vi "4Pi Focus Lock_v1.vi"() -> ()   [LabVIEW 2016]
uses:
  4Pi Focus Lock Controls/4Pi Focus Lock - Notifier Type.ctl
  4Pi Focus Lock Controls/4Pi Focus Lock - Actions.ctl
  <vilib>/vision/Image Controls.llb/IMAQ Image.ctl
  Hardware Configuration/Hardware Configuration Controls/Device Type.ctl
  Hardware Configuration/Hardware Configuration Controls/Device Function.ctl
  Device Library/Cameras/Camera Controls/Generic Camera ROI.ctl
  Device Library/Cameras/Camera Controls/Generic Camera Actions.ctl
  Device Library/Stages/Stages Controls/Stage Actions.ctl
  <vilib>/addons/control/pid/pid.llb/PID (DBL).vi
  <vilib>/vision/NI_Vision_Development_Module.lvlib
  <vilib>/addons/control/pid/NI_PID_pid.lvlib
panel:
  in  "Z Drift Threshold (µm)":dbl=2.0
  in  "Z Move Limit (µm)":dbl=2.0
  out "Z Move":bool
  in  "Update Scale Factor":dbl=2.0
  out "dz (µm)":dbl format="%.2f"
  out "dt (s)":dbl format="%.3f"
  out "Measured Z (µm)":dbl=1.0 format="%.3g"
  out "Target Z (µm)":dbl=1.0 format="%.3g"
  out "Stage Position (µm)":dbl=1.0 format="%.2g"
  in  "Quit":bool
  in  "Sample Z Step No.":u32=2
  in  "Sample Z Step Size (µm)":dbl=2.0
  in  "D (Derivative)":dbl
  in  "I (Integral)":dbl
  in  "P (Proportional)":dbl=2.0
  in  "Set Camera ROI":bool
  out "Z Target and Fit Value (µm)":T1(graph)
  in  "Start Lock":bool
  # "PID Control Values"
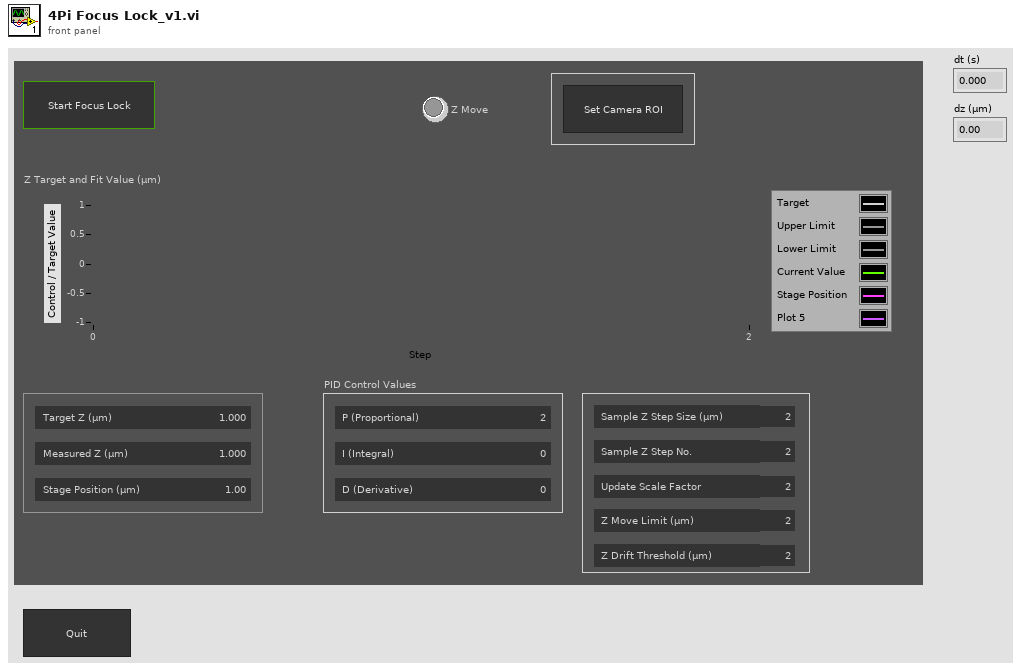
[diagram p1: front panel]
types:
  T1 = cluster{"Target 01":dbl, dbl, dbl, "Current 01":dbl, "Stage Position":dbl}
  T2 = typedef "4Pi Focus Lock - Actions.ctl" = enum16{"Idle", "Start Lock", "Restart Lock", "Get Target Position", "Get Ref Stack", "Cal Ref FFT", "Move To Init Z", "Start Primary Camera", "Get Current Position", "Get Current XY Position", "Get Current Position 1", "Get Actual Position", "Check Drift", "Move Z", "Update Plots", "Delay", "Abort", "Exit Loop", "Quit"}
  T3 = typedef "4Pi Focus Lock - Notifier Type.ctl" = cluster{"Actions":T2, "Z Drift Threshold":dbl, "Z Stage Move Limit (µm)":dbl, "Abort If Error":bool, "Z Correction Active":bool, "PID Values":dbl[], "Running?":bool, "Update Delay (ms)":i32, "Z Step Size (µm)":dbl, "Z Step No.":u32, "No. of Frames":u32, "Ref Stack (SGL)":T4[], "Cur Image (SGL)":T4, "CC Image (SGL) ":T4, "Sample Z (µm)":dbl[], "Initial Z Position (µm)":dbl, "Ref FFT Stack (CSG)":T4[], "Tmp Image FFT (CSG) ":T4[], "CC Image Max (SGL)":T4}
  T4 = typedef "IMAQ Image.ctl" = refnum<image>
  T5 = typedef "Image Type" = u32
  T6 = typedef "Device Function.ctl" = enum16{"Primary", "Secondary", "Overview", "Wide Field Drift Correction", "642 nm Excitation", "560 nm Excitation", "940 nm Excitation", "546 nm Excitation", "488 nm Excitation", "405 nm Excitation", "Objective Drift Correction", "4Pi Focus Lock", "4Pi Objective Lock", "Objective XY", "Objective Z", "Sample XY", "Sample Coarse Z", "Sample Z", "4Pi Lower", "4Pi Upper", "Em Small", "Em Large", "Ex Small", "Ex Large", "Mojo", "Adj Cavity", "Line Scanning", "Alert"}
  T7 = typedef "Device Type.ctl" = enum16{"AOTF", "Camera", "Deformable Mirror", "Laser", "Flip Mirror", "Shutter", "Stage", "Waveform", "FPGA", "Email"}
  T8 = typedef "Stage Actions.ctl" = enum16{"Get Position", "MVR", "MOVE", "HALT", "ONTARGET", "ERROR", "REFERENCE", "INIT", "VELOCITY", "STATUS", "EXIT", "HOME", "ZEROPOS", "NANOPOS", "ANALOG", "QUIT"}
  T9 = typedef "Generic Camera Actions.ctl" = enum16{"Status", "Live Preview", "Capture", "Abort", "Set Exposure Time (s)", "Get Exposure Time (s)", "Record Settings", "Set ROI", "Get ROI", "Defect Correction On/Off", "Cooler On/Off", "Fan On/Off", "Quit"}
  T10 = typedef "Generic Camera ROI.ctl" = cluster{"H_Offset":u16, "V_Offset":u16, "H_Width":u16, "V_Width":u16}
  T11 = typedef "Stage Status.ctl" = enum16{"Error", "Abort", "Busy", "On Target"}
  T12 = cluster{"PID Values[0]":dbl, "PID Values[1]":dbl, "PID Values[2]":dbl}
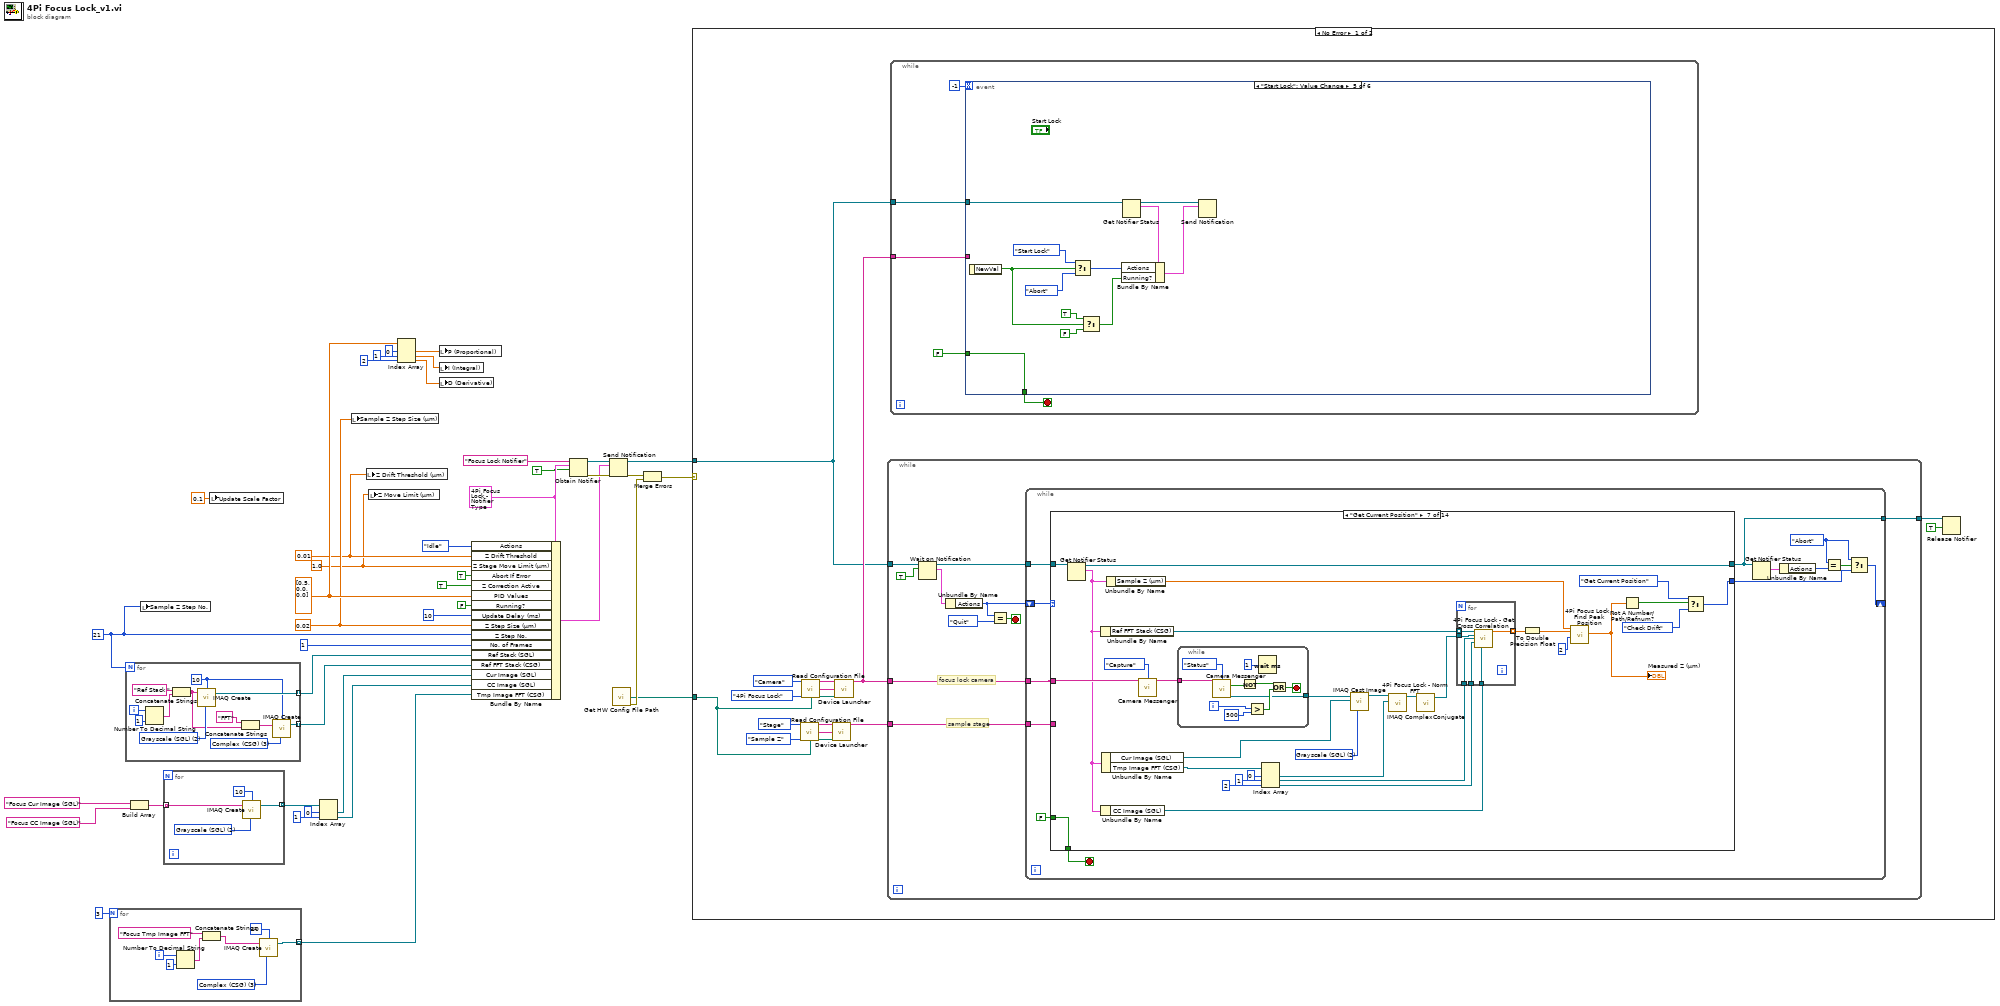
[diagram p0: block diagram]
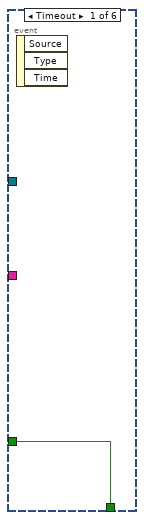
[diagram p2: hidden frame]
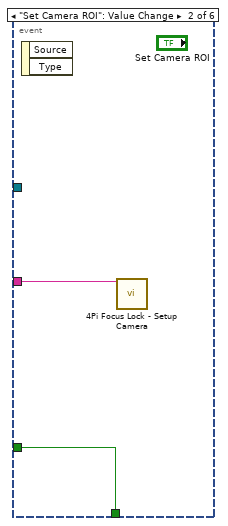
[diagram p3: hidden frame]
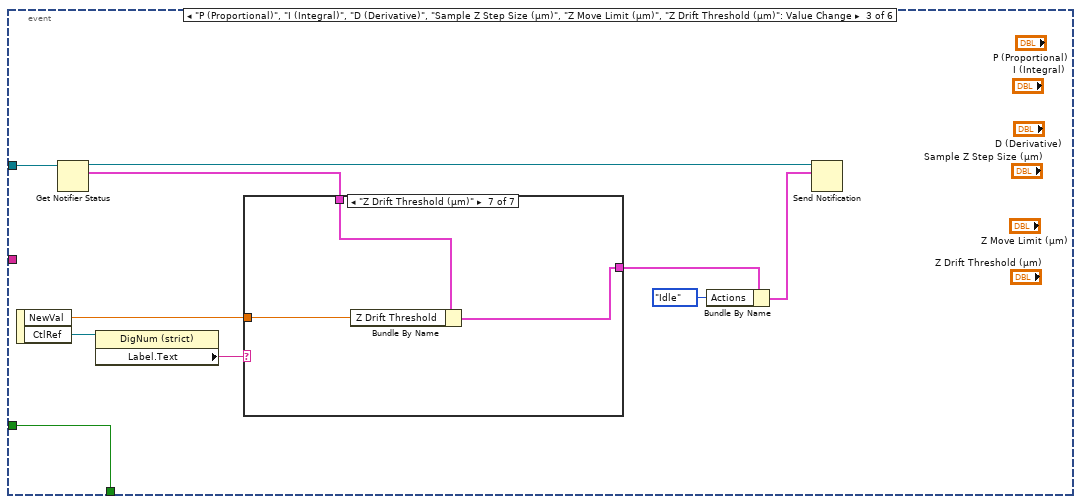
[diagram p4: hidden frame]
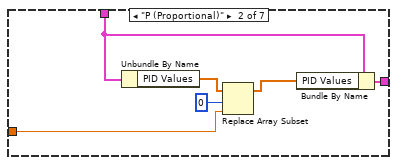
[diagram p6: hidden frame]
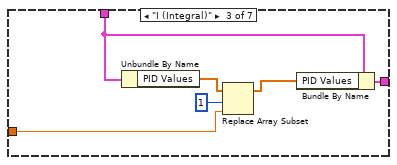
[diagram p7: hidden frame]
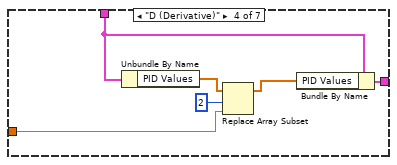
[diagram p8: hidden frame]
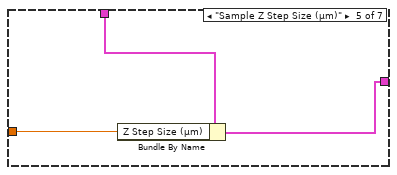
[diagram p9: hidden frame]
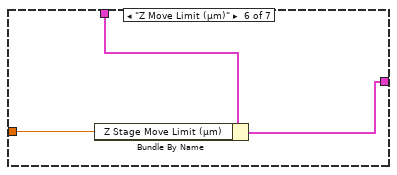
[diagram p10: hidden frame]
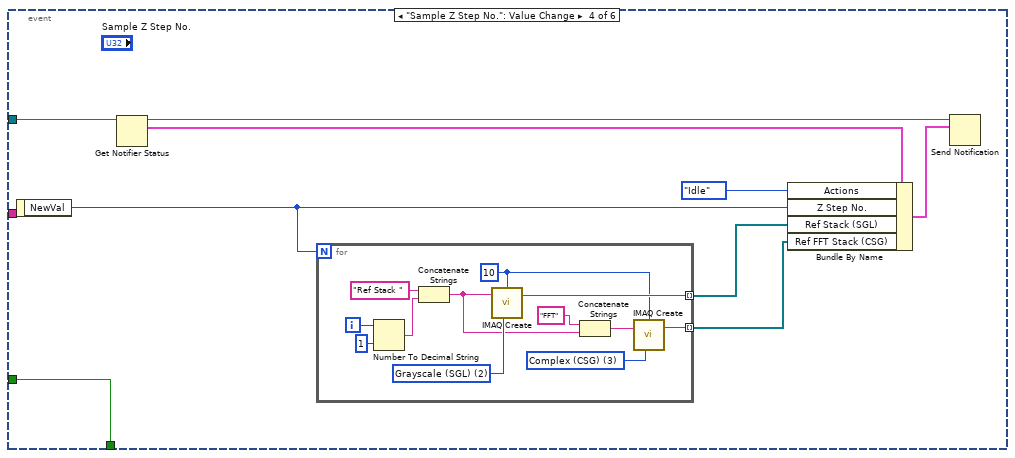
[diagram p11: hidden frame]
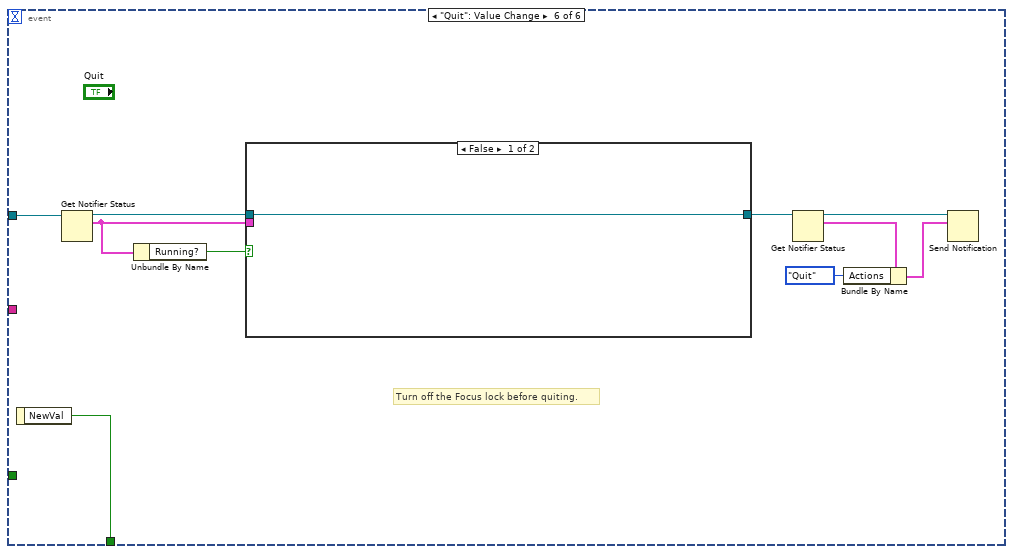
[diagram p12: hidden frame]
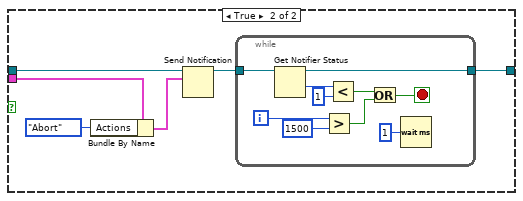
[diagram p13: hidden frame]
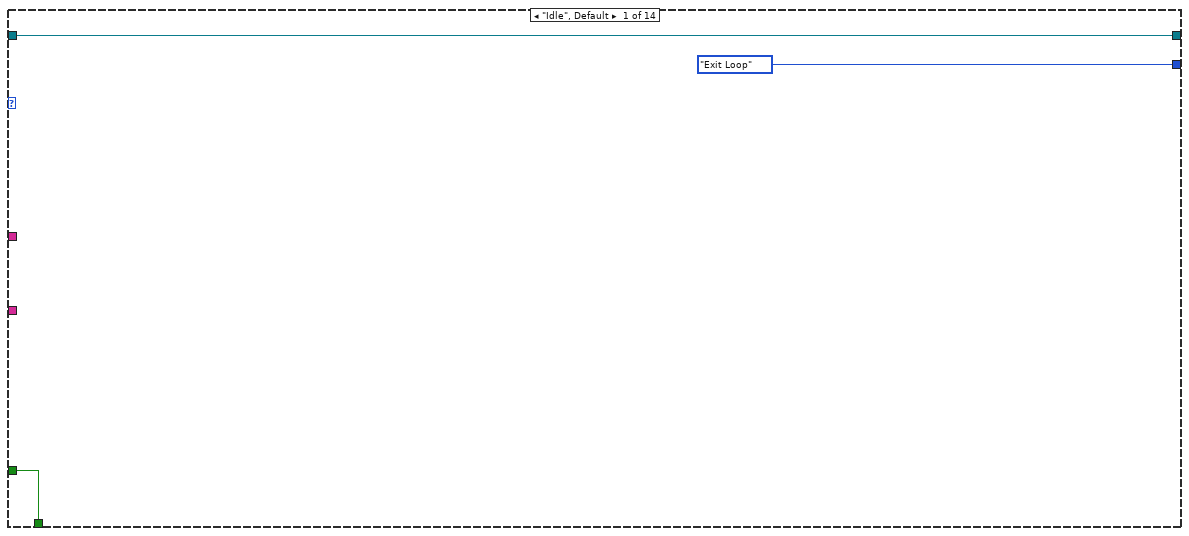
[diagram p14: hidden frame]
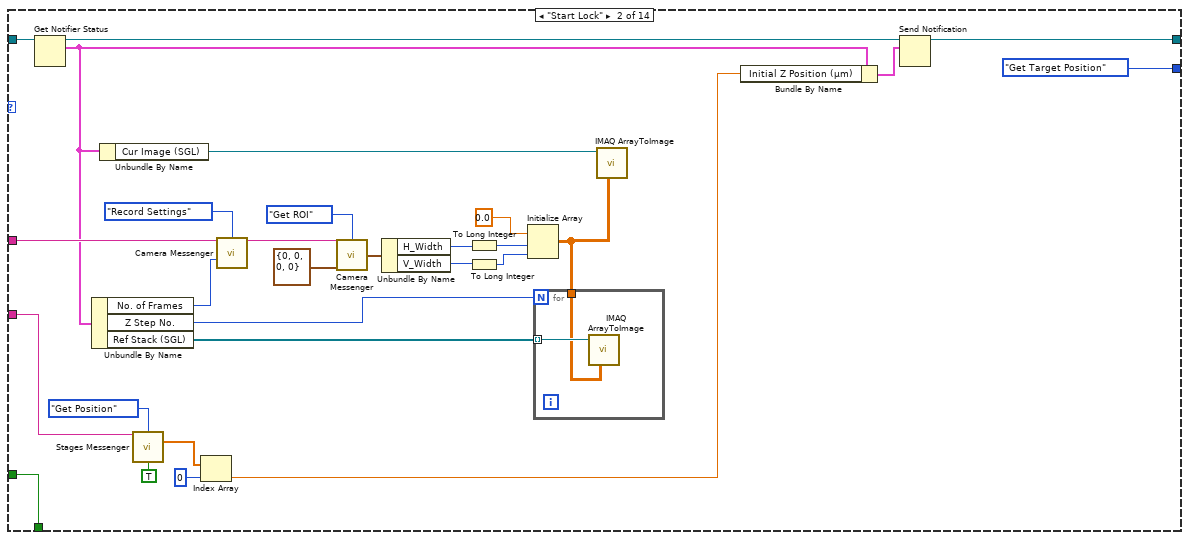
[diagram p15: hidden frame]
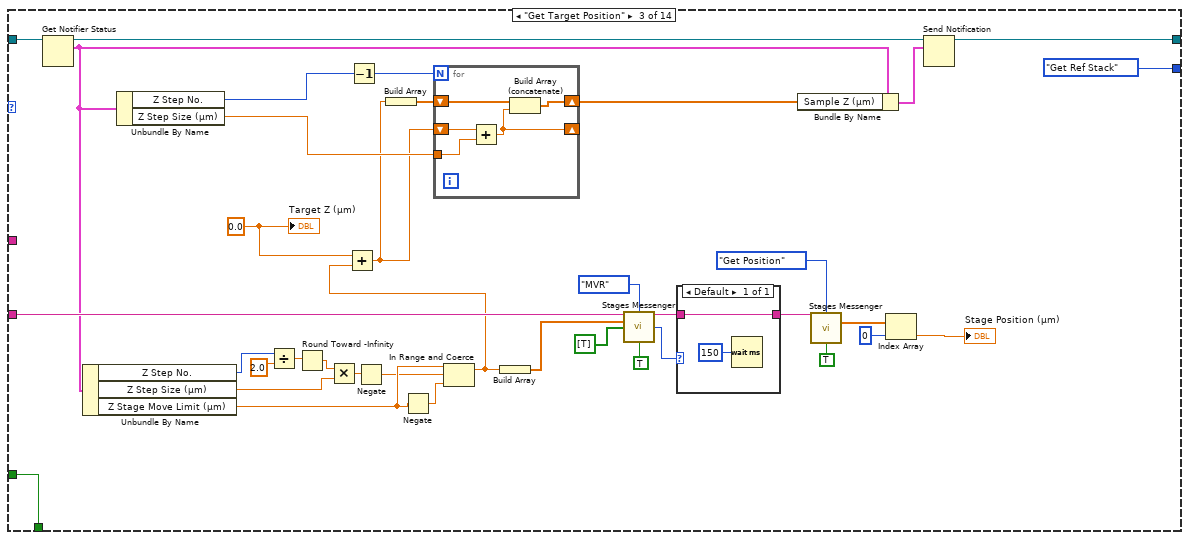
[diagram p16: hidden frame]
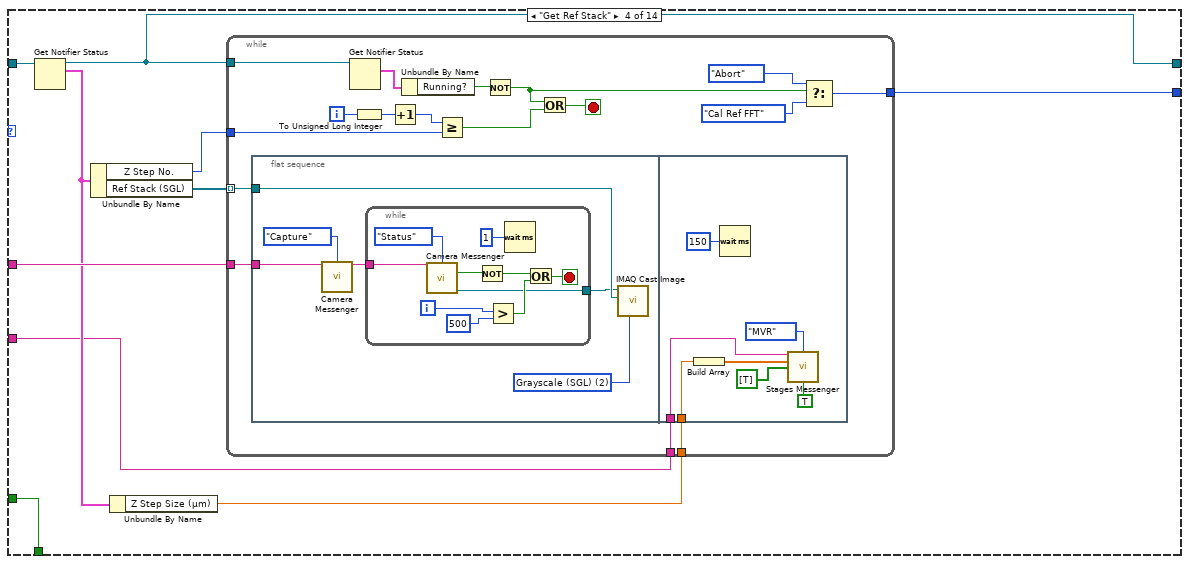
[diagram p17: hidden frame]
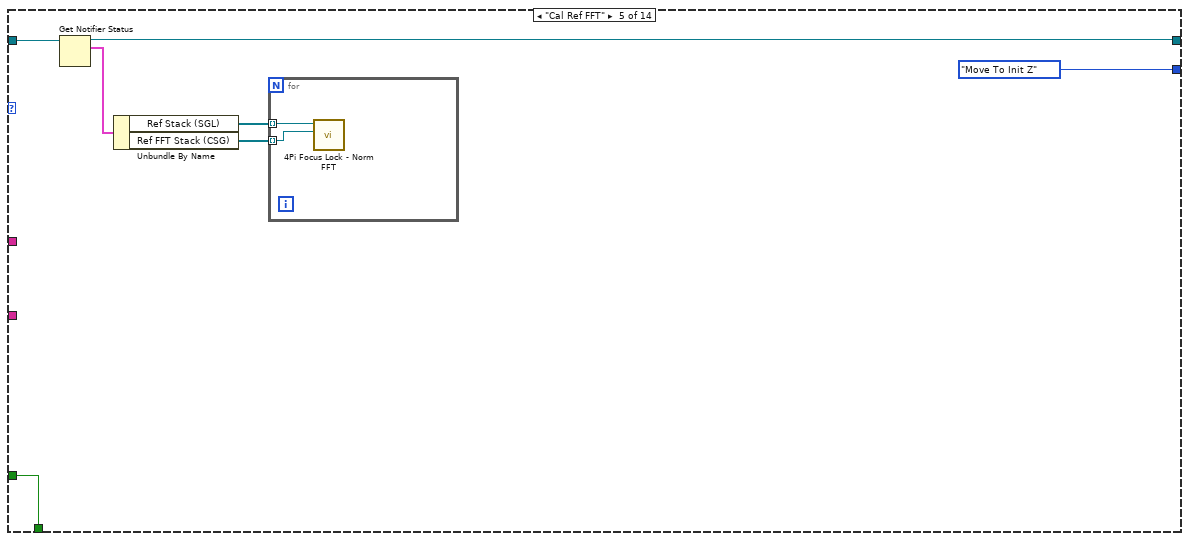
[diagram p18: hidden frame]
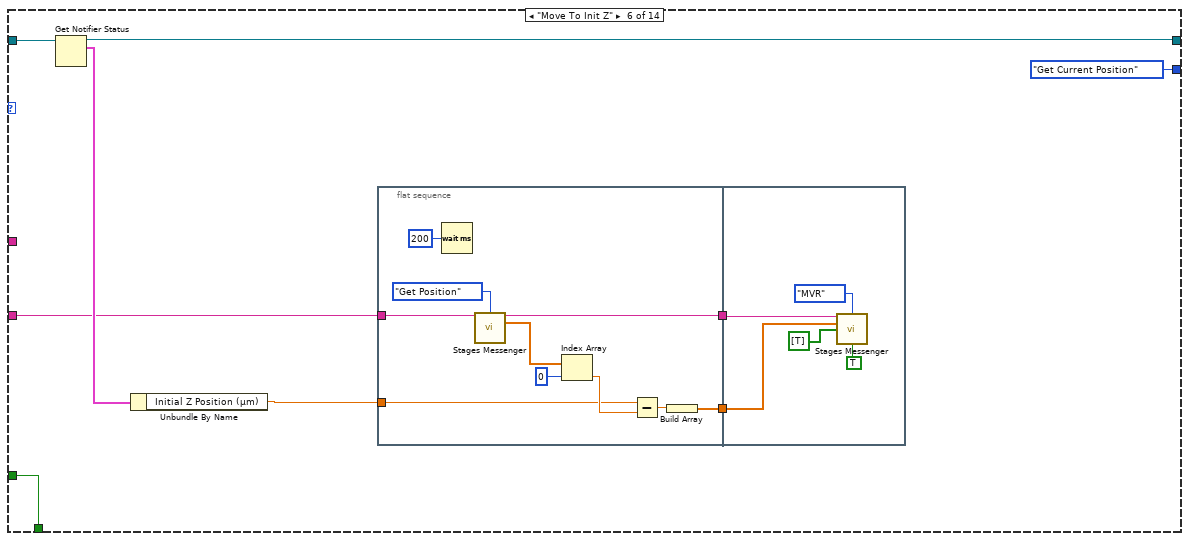
[diagram p19: hidden frame]
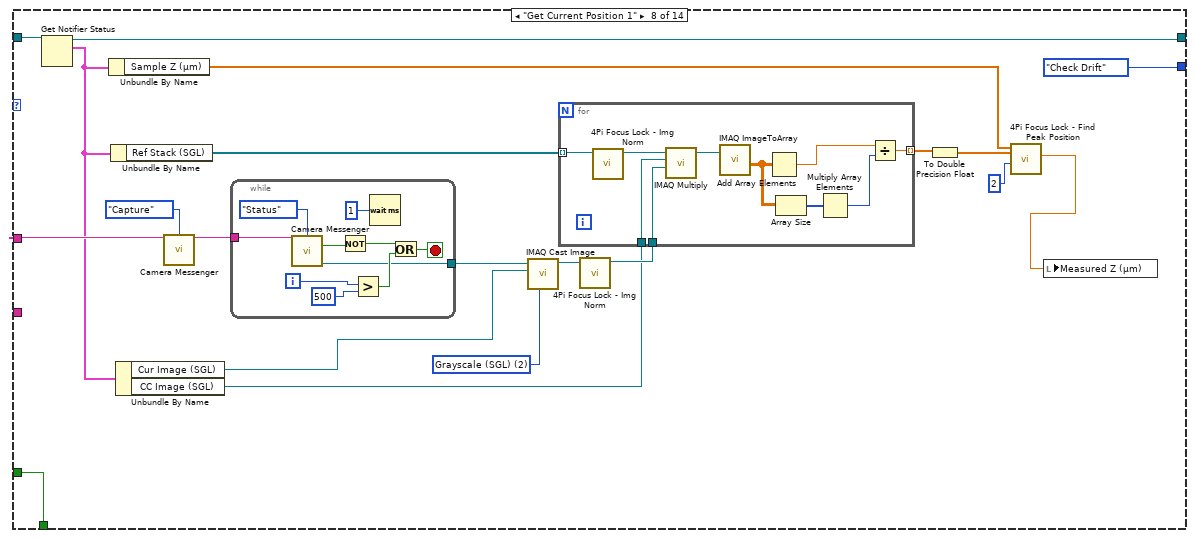
[diagram p20: hidden frame]
diagram:
  w19 = u32 21 ("Z Step No.")
  w26 = 0.02 ("Z Step Size (µm)")
  w30 = dbl[] [0.5, 0.0, 0.0] ("PID Values")
  w6 = 1.0 ("Z Stage Move Limit (µm)")
  w7 = 0.01 ("Z Drift Threshold")
  w9 = T3 {"Actions"=enum."Idle", "Z Drift Threshold"=0.05, "Z Stage Move Limit (µm)"=1.0, "Abort If Error"=FALSE, "Z Correction Active"=FALSE, "PID Values"=[], "Running?"=FALSE, "Update Delay (ms)"=0, "Z Step Size (µm)"=2.0, "Z Step No."=2, "No. of Frames"=0, "Ref Stack (SGL)"=[], "Cur Image (SGL)"=refnum, "CC Image (SGL) "=refnum, "Sample Z (µm)"=[], "Initial Z Position (µm)"=0.0, "Ref FFT Stack (CSG)"=[], "Tmp Image FFT (CSG) "=[], "CC Image Max (SGL)"=refnum} ("4Pi Focus Lock")
  n1 = for {
    N: 3 -> [_]
    tunnel: [w47] -> w1 mode=indexing
    i -> [w43]
    w48 = T5 3 items=["Grayscale (U8)", "Grayscale (I16)", "Grayscale (SGL)", "Complex (CSG)", "RGB (U32)", "HSL (U32)", "RGB (U64)", "Grayscale (U16)"] ("Image Type")
    n2 = Number To Decimal String(number=w43, width (-)=i16 1) -> (decimal integer string=w46:string)
    n3 = Concatenate Strings("Focus Tmp Image FFT" ("Image Name"), w46) -> (w42:string)
    n4 = call "IMAQ Create"("Border Size"=10, "Image Name"=w42, "Image Type"=w48) -> ("New Image"=w47:T4)  [unwired: 2 in, 1 out]
  }
  n5 = for {
    N: w19 -> [_]
    tunnel: [w61] -> w18 mode=indexing
    tunnel: [w50] -> w3 mode=indexing
    i -> [w60]
    w55 = T5 3 items=["Grayscale (U8)", "Grayscale (I16)", "Grayscale (SGL)", "Complex (CSG)", "RGB (U32)", "HSL (U32)", "RGB (U64)", "Grayscale (U16)"] ("Image Type")
    w56 = T5 2 items=["Grayscale (U8)", "Grayscale (I16)", "Grayscale (SGL)", "Complex (CSG)", "RGB (U32)", "HSL (U32)", "RGB (U64)", "Grayscale (U16)"] ("Image Type")
    w52 = 10 ("Border Size")
    n6 = Number To Decimal String(number=w60, width (-)=i16 1) -> (decimal integer string=w58:string)
    n7 = Concatenate Strings("Ref Stack " ("string"), w58) -> (w51:string)
    n8 = call "IMAQ Create"("Border Size"=w52, "Image Name"=w51, "Image Type"=w56) -> ("New Image"=w61:T4)  [unwired: 2 in, 1 out]
    n9 = Concatenate Strings("FFT" ("string"), w51) -> (w54:string)
    n10 = call "IMAQ Create"("Border Size"=w52, "Image Name"=w54, "Image Type"=w55) -> ("New Image"=w50:T4)  [unwired: 2 in, 1 out]
  }
  n11 = Build Array("Focus Cur Image (SGL)" ("Image Name"), "Focus CC Image (SGL)" ("Image Name")) -> (w13:string[])
  n12 = local write "Sample Z Step No."(w19) -> ()
  n13 = for {
    tunnel: w13 -> [w63] mode=indexing
    tunnel: [w62] -> w12 mode=indexing
    w64 = T5 2 items=["Grayscale (U8)", "Grayscale (I16)", "Grayscale (SGL)", "Complex (CSG)", "RGB (U32)", "HSL (U32)", "RGB (U64)", "Grayscale (U16)"] ("Image Type")
    n14 = call "IMAQ Create"("Border Size"=10, "Image Name"=w63, "Image Type"=w64) -> ("New Image"=w62:T4)  [unwired: 2 in, 1 out]
  }
  n15 = local write "Update Scale Factor"(0.1 ("Update Scale Factor")) -> ()
  n16 = Index Array(array=w12, index #1=0 ("index"), index #2=1 ("index")) -> (element #1=w11:T4, element #2=w10:T4)
  n17 = local write "Sample Z Step Size (µm)"(w26) -> ()
  n18 = local write "Z Drift Threshold (µm)"(w7) -> ()
  n19 = local write "Z Move Limit (µm)"(w6) -> ()
  n20 = Index Array(array=w30, index #1=0 ("index"), index #2=1 ("index"), index #3=2 ("index")) -> (element #1=w29:dbl, element #2=w28:dbl, element #3=w27:dbl)
  n21 = local write "P (Proportional)"(w29) -> ()
  n22 = local write "I (Integral)"(w28) -> ()
  n23 = local write "D (Derivative)"(w27) -> ()
  n24 = Bundle By Name(cluster=w9, "Actions"=4Pi_Focus_Lock_-_Actions."Idle", "Z Drift Threshold"=w7, "Z Stage Move Limit (µm)"=w6, "Abort If Error"=TRUE, "Z Correction Active"=TRUE, "PID Values"=w30, "Running?"=FALSE, "Update Delay (ms)"=10, "Z Step Size (µm)"=w26, "Z Step No."=w19, "No. of Frames"=u32 1, "Ref Stack (SGL)"=w18, "Ref FFT Stack (CSG)"=w3, "Cur Image (SGL)"=w11, "CC Image (SGL)"=w10, "Tmp Image FFT (CSG)"=w1) -> (w4:T3)
  n25 = Obtain Notifier(name (unnamed)="Focus Lock Notifier", notification data type=w9, create if not found? (T)=TRUE) -> (notifier out=w35:refnum<notifier>, error out=w34:errorcluster)  [unwired: 1 in, 1 out]
  n26 = Send Notification(notification=w4, notifier=w35, error in (no error)=w34) -> (notifier out=w21:refnum<notifier>, error out=w25:errorcluster)
  n27 = call "Get HW Config File Path.vi"() -> ("File Path"=w23:path, "Error"=w24:errorcluster)  [unwired: 14 in]
  n28 = Merge Errors(w25, w24) -> (w22:errorcluster)
  n29 = case shown="No Error" w22 {
    tunnel: w23 -> [w66 _]
    tunnel: w21 -> [w69 _]
    frame No Error {
      n30 = call "Read Configuration File.vi"("Device Type"=Device_Type."Stage", "Device Function"=Device_Function."Sample Z", "Config File Path"=w66) -> ("Unique Notifier Name"=w76:string, "Device Ports/IDs/Channels"=w74:string[], "Device Engine Path"=w73:path)  [unwired: 9 in, 1 out]
      n31 = call "Read Configuration File.vi"("Device Type"=Device_Type."Camera", "Device Function"=Device_Function."4Pi Focus Lock", "Config File Path"=w66) -> ("Unique Notifier Name"=w81:string, "Device Ports/IDs/Channels"=w80:string[], "Device Engine Path"=w79:path)  [unwired: 9 in, 1 out]
      n32 = call "Device Launcher.vi"("Notifier Name"=w76, "Device Ports/IDs/Channels"=w74, "Device Engine Path"=w73) -> ("Notifier Name"=w71:string)  [unwired: 11 in, 1 out]
      n33 = call "Device Launcher.vi"("Notifier Name"=w81, "Device Ports/IDs/Channels"=w80, "Device Engine Path"=w79) -> ("Notifier Name"=w70:string)  [unwired: 11 in, 1 out]
      n34 = while {
        tunnel: w69 -> [w197]
        tunnel: w70 -> [w191]
        tunnel: w71 -> [w190]
        tunnel: [w188] -> w67
        stop <- w193 stop-if-true
        # "sample stage"
        # "focus lock camera"
        n35 = Wait on Notification(notifier=w197, ignore previous (F)=TRUE) -> (notifier out=w189:refnum<notifier>, notification=w195:T3)  [unwired: 2 in, 2 out]
        n36 = Unbundle By Name(w195) -> ("Actions"=w192:T2)
        n37 = Equal?(x=w192, y=4Pi_Focus_Lock_-_Actions."Quit") -> (x = y?=w193:bool)
        n38 = while {
          tunnel: w191 -> [w209]
          tunnel: w190 -> [w208]
          tunnel: w189 -> [w207]
          shift-right: [w201] -> _
          shift-left: w192 -> [w210]
          tunnel: [w198] -> w188
          stop <- w200 stop-if-true
          w203 = 4Pi_Focus_Lock_-_Actions."Abort" ("y")
          n39 = case shown="\"Get Current Position\"" w210 {
            tunnel: w209 -> [_ w233 _ w297 _ _ w401 w437 _ _ _ w519 _ _]
            tunnel: w208 -> [_ w222 w276 w289 _ w351 _ _ _ w483 w502 _ _ _]
            tunnel: w207 -> [w211 w235 w277 w298 w344 w356 w400 w436 w470 w488 w512 w520 w527 w530]
            tunnel: [4Pi_Focus_Lock_-_Actions."Exit Loop" ("y") 4Pi_Focus_Lock_-_Actions."Get Target Position" ("y") 4Pi_Focus_Lock_-_Actions."Get Ref Stack" ("y") w290 4Pi_Focus_Lock_-_Actions."Move To Init Z" ("y") 4Pi_Focus_Lock_-_Actions."Get Current Position" ("y") w381 4Pi_Focus_Lock_-_Actions."Check Drift" ("y") 4Pi_Focus_Lock_-_Actions."Move Z" ("y") w473 4Pi_Focus_Lock_-_Actions."Get Current Position" ("y") 4Pi_Focus_Lock_-_Actions."Exit Loop" ("y") 4Pi_Focus_Lock_-_Actions."Exit Loop" ("y") 4Pi_Focus_Lock_-_Actions."Quit" ("y")] -> w202
            tunnel: [w211 w216 w264 w292 w341 w354 w394 w430 w460 w481 w500 w516 w527 w530] -> w198
            tunnel: [w212 w215 w263 w291 w339 w352 w393 w429 w459 w480 w499 w515 TRUE TRUE] -> w200
            tunnel: FALSE -> [w212 w215 w263 w291 w339 w352 w393 w429 w459 w480 w499 w515 _ _]
            frame "Idle", Default {
            }
            frame "Start Lock" {
              n40 = Get Notifier Status(notifier=w235) -> (notifier out=w218:refnum<notifier>, current notification=w221:T3)  [unwired: 1 in, 3 out]
              n41 = Unbundle By Name(w221) -> ("No. of Frames"=w230:u32, "Z Step No."=w229:u32, "Ref Stack (SGL)"=w228:T4[])
              n42 = Unbundle By Name(w221) -> ("Cur Image (SGL)"=w226:T4)
              n43 = call "Stages Messenger.vi"("Stage Notifier Name"=w222, "Actions"=Stage_Actions."Get Position", "Exit While Busy?"=TRUE) -> ("Positions"=w223:dbl[])  [unwired: 9 in, 3 out]
              n44 = Index Array(array=w223, index=0) -> (element=w220:dbl)
              n45 = call "Camera Messenger.vi"("Notifier Name"=w233, "General Camera Actions"=Generic_Camera_Actions."Record Settings", "No. of Frames"=w230) -> ("Notifier Name Dup"=w231:string)  [unwired: 7 in, 5 out]
              n46 = call "Camera Messenger.vi"("Notifier Name"=w231, "General Camera Actions"=Generic_Camera_Actions."Get ROI", "Camera ROI"=T10 {"H_Offset"=0, "V_Offset"=0, "H_Width"=0, "V_Width"=0} ("General Camera ROI")) -> ("Camera ROI"=w240:T10)  [unwired: 7 in, 5 out]
              n47 = Unbundle By Name(w240) -> ("H_Width"=w239:u16, "V_Width"=w237:u16)
              n48 = To Long Integer(number=w239) -> (32bit integer=w238:i32)
              n49 = To Long Integer(number=w237) -> (32bit integer=w236:i32)
              n50 = Initialize Array(sgl 0.0 ("element"), w238, w236) -> (w227:sgl[][])
              n51 = for {
                N: w229 -> [_]
                tunnel: w227 -> [w243]
                tunnel: w228 -> [w244] mode=indexing
                n52 = call "IMAQ ArrayToImage"("Image Pixels (Float)"=w243, "Image"=w244) -> ()  [unwired: 8 in, 2 out]
              }
              n53 = call "IMAQ ArrayToImage"("Image Pixels (Float)"=w227, "Image"=w226) -> ()  [unwired: 8 in, 2 out]
              n54 = Bundle By Name(cluster=w221, "Initial Z Position (µm)"=w220) -> (w219:T3)
              n55 = Send Notification(notification=w219, notifier=w218) -> (notifier out=w216:refnum<notifier>)  [unwired: 1 in, 1 out]
            }
            frame "Get Target Position" {
              w270 = 0.0 ("Target Z (µm)")
              n56 = Get Notifier Status(notifier=w277) -> (notifier out=w268:refnum<notifier>, current notification=w273:T3)  [unwired: 1 in, 3 out]
              n57 = Unbundle By Name(w273) -> ("Z Step No."=w262:u32, "Z Step Size (µm)"=w261:dbl, "Z Stage Move Limit (µm)"=w259:dbl)
              n58 = Unbundle By Name(w273) -> ("Z Step No."=w254:u32, "Z Step Size (µm)"=w271:dbl)
              n59 = Divide(x=w262, y=2.0) -> (x/y=w252:dbl)
              n60 = Round Toward -Infinity(1:w252) -> (0:w251:dbl)
              n61 = Multiply(x=w251, y=w261) -> (x*y=w256:dbl)
              n62 = Decrement(x=w254) -> (x-1=w253:u32)
              n63 = Negate(x=w256) -> (-x=w255:dbl)
              n64 = Negate(x=w259) -> (-x=w260:dbl)
              n65 = In Range and Coerce(upper limit=w259, x=w255, lower limit=w260) -> (coerced(x)=w257:dbl)  [unwired: 1 out]
              n66 = Add(x=w270, y=w257) -> (x+y=w258:dbl)
              n67 = Build Array(w258) -> (w272:dbl[])
              n68 = for {
                N: w253 -> [_]
                tunnel: w271 -> [w286]
                shift-right: [w287] -> w269
                shift-left: w272 -> [w288]
                shift-right: [w284] -> _
                shift-left: w258 -> [w285]
                n69 = Add(x=w285, y=w286) -> (x+y=w284:dbl)
                n70 = Build Array (concatenate)(w288, w284) -> (w287:dbl[])
              }
              n71 = Build Array(w257) -> (w274:dbl[])
              n72 = call "Stages Messenger.vi"("Stage Notifier Name"=w276, "Actions"=Stage_Actions."MVR", "Setpoint"=w274, "Axis"=bool[] [TRUE], "Exit While Busy?"=TRUE) -> ("Stage Notifier Name (Dup)"=w249:string, "Status"=w250:T11)  [unwired: 7 in, 2 out]
              n73 = case shown="Default" w250 {
                tunnel: [w282] -> w248
                tunnel: w249 -> [w282]
                frame Default {
                  n74 = Wait (ms)(milliseconds to wait=u32 150) -> ()  [unwired: 1 out]
                }
              }
              n75 = Bundle By Name(cluster=w273, "Sample Z (µm)"=w269) -> (w267:T3)
              n76 = call "Stages Messenger.vi"("Stage Notifier Name"=w248, "Actions"=Stage_Actions."Get Position", "Exit While Busy?"=TRUE) -> ("Positions"=w246:dbl[])  [unwired: 9 in, 3 out]
              n77 = Index Array(array=w246, index=0) -> (element=→"Stage Position (µm)":dbl)
              n78 = Send Notification(notification=w267, notifier=w268) -> (notifier out=w264:refnum<notifier>)  [unwired: 1 in, 1 out]
              "Target Z (µm)" <- w270
            }
            frame "Get Ref Stack" {
              n79 = Get Notifier Status(notifier=w298) -> (notifier out=w292:refnum<notifier>, current notification=w296:T3)  [unwired: 1 in, 3 out]
              n80 = Unbundle By Name(w296) -> ("Z Step No."=w295:u32, "Ref Stack (SGL)"=w294:T4[])
              n81 = Unbundle By Name(w296) -> ("Z Step Size (µm)"=w293:dbl)
              n82 = while {
                tunnel: w297 -> [w315]
                tunnel: w295 -> [w312]
                tunnel: w292 -> [w314]
                tunnel: [w302] -> w290
                tunnel: w294 -> [w301] mode=indexing
                tunnel: w293 -> [w300]
                tunnel: w289 -> [w299]
                i -> [w311]
                stop <- w307 stop-if-true
                n83 = flat-sequence {
                  tunnel: w315 -> [w321]
                  tunnel: w301 -> [w318]
                  tunnel: w300 -> [w333]
                  tunnel: w299 -> [w332]
                  frame #0 {
                    w319 = T5 2 items=["Grayscale (U8)", "Grayscale (I16)", "Grayscale (SGL)", "Complex (CSG)", "RGB (U32)", "HSL (U32)", "RGB (U64)", "Grayscale (U16)"] ("Image Type")
                    n84 = call "Camera Messenger.vi"("Notifier Name"=w321, "General Camera Actions"=Generic_Camera_Actions."Capture") -> ("Notifier Name Dup"=w317:string)  [unwired: 8 in, 5 out]
                    n85 = while {
                      tunnel: w317 -> [w331]
                      tunnel: [w324] -> w316
                      i -> [w327]
                      stop <- w325 stop-if-true
                      n86 = call "Camera Messenger.vi"("Notifier Name"=w331, "General Camera Actions"=Generic_Camera_Actions."Status") -> ("Running?"=w323:bool, "Image Ref"=w324:T4)  [unwired: 8 in, 4 out]
                      n87 = Not(x=w323) -> (.not. x?=w322:bool)
                      n88 = Greater?(x=w327, y=500) -> (0:w329:bool)
                      n89 = Wait (ms)(milliseconds to wait=u32 1) -> ()  [unwired: 1 out]
                      n90 = Or(x=w322, y=w329) -> (x .or. y?=w325:bool)
                    }
                    n91 = call "IMAQ Cast Image"("Image Type"=w319, "Image Dst"=w318, "Image Src"=w316) -> ()  [unwired: 7 in, 2 out]
                  }
                  frame #1 {
                    n92 = Build Array(w333) -> (w337:dbl[])
                    n93 = Wait (ms)(milliseconds to wait=u32 150) -> ()  [unwired: 1 out]
                    n94 = call "Stages Messenger.vi"("Stage Notifier Name"=w332, "Actions"=Stage_Actions."MVR", "Setpoint"=w337, "Axis"=bool[] [TRUE], "Exit While Busy?"=TRUE) -> ()  [unwired: 7 in, 4 out]
                  }
                }
                n95 = Get Notifier Status(notifier=w314) -> (current notification=w306:T3)  [unwired: 1 in, 4 out]
                n96 = To Unsigned Long Integer(number=w311) -> (unsigned 32bit integer=w310:u32)
                n97 = Increment(x=w310) -> (x+1=w313:u32)
                n98 = Unbundle By Name(w306) -> ("Running?"=w309:bool)
                n99 = Greater Or Equal?(x=w313, y=w312) -> (x >= y?=w308:bool)
                n100 = Not(x=w309) -> (.not. x?=w305:bool)
                n101 = Or(x=w305, y=w308) -> (x .or. y?=w307:bool)
                n102 = Select(t=4Pi_Focus_Lock_-_Actions."Abort", s=w305, f=4Pi_Focus_Lock_-_Actions."Cal Ref FFT" ("y")) -> (s? t:f=w302:T2)
              }
            }
            frame "Cal Ref FFT" {
              n103 = Get Notifier Status(notifier=w344) -> (notifier out=w341:refnum<notifier>, current notification=w345:T3)  [unwired: 1 in, 3 out]
              n104 = Unbundle By Name(w345) -> ("Ref Stack (SGL)"=w342:T4[], "Ref FFT Stack (CSG)"=w343:T4[])
              n105 = for {
                tunnel: w343 -> [w346] mode=indexing
                tunnel: w342 -> [w347] mode=indexing
                n106 = call "4Pi Focus Lock - Norm FFT.vi"("FFT Image Dst"=w346, "Image In"=w347) -> ()  [unwired: 8 in, 2 out]
              }
            }
            frame "Move To Init Z" {
              n107 = Get Notifier Status(notifier=w356) -> (notifier out=w354:refnum<notifier>, current notification=w355:T3)  [unwired: 1 in, 3 out]
              n108 = Unbundle By Name(w355) -> ("Initial Z Position (µm)"=w349:dbl)
              n109 = flat-sequence {
                tunnel: w351 -> [w364]
                tunnel: [w363] -> w350
                tunnel: w349 -> [w359]
                tunnel: [w357] -> w348
                tunnel: w350 -> [w368]
                tunnel: w348 -> [w367]
                frame #0 {
                  n110 = Wait (ms)(milliseconds to wait=u32 200) -> ()  [unwired: 1 out]
                  n111 = call "Stages Messenger.vi"("Stage Notifier Name"=w364, "Actions"=Stage_Actions."Get Position") -> ("Stage Notifier Name (Dup)"=w363:string, "Positions"=w361:dbl[])  [unwired: 10 in, 2 out]
                  n112 = Index Array(array=w361, index=0) -> (element=w360:dbl)
                  n113 = Subtract(x=w359, y=w360) -> (x-y=w358:dbl)
                  n114 = Build Array(w358) -> (w357:dbl[])
                }
                frame #1 {
                  n115 = call "Stages Messenger.vi"("Stage Notifier Name"=w368, "Actions"=Stage_Actions."MVR", "Setpoint"=w367, "Axis"=bool[] [TRUE], "Exit While Busy?"=TRUE) -> ()  [unwired: 7 in, 4 out]
                }
              }
            }
            frame "Get Current Position" {
              w399 = T5 2 items=["Grayscale (U8)", "Grayscale (I16)", "Grayscale (SGL)", "Complex (CSG)", "RGB (U32)", "HSL (U32)", "RGB (U64)", "Grayscale (U16)"] ("Image Type")
              n116 = Get Notifier Status(notifier=w400) -> (notifier out=w394:refnum<notifier>, current notification=w373:T3)  [unwired: 1 in, 3 out]
              n117 = Unbundle By Name(w373) -> ("Ref FFT Stack (CSG)"=w389:T4[])
              n118 = Unbundle By Name(w373) -> ("CC Image (SGL)"=w372:T4)
              n119 = Unbundle By Name(w373) -> ("Cur Image (SGL)"=w390:T4, "Tmp Image FFT (CSG)"=w377:T4[])
              n120 = Unbundle By Name(w373) -> ("Sample Z (µm)"=w396:dbl[])
              n121 = call "Camera Messenger.vi"("Notifier Name"=w401, "General Camera Actions"=Generic_Camera_Actions."Capture") -> ("Notifier Name Dup"=w392:string)  [unwired: 8 in, 5 out]
              n122 = while {
                tunnel: w392 -> [w418]
                tunnel: [w412] -> w391
                i -> [w414]
                stop <- w413 stop-if-true
                n123 = call "Camera Messenger.vi"("Notifier Name"=w418, "General Camera Actions"=Generic_Camera_Actions."Status") -> ("Running?"=w410:bool, "Image Ref"=w412:T4)  [unwired: 8 in, 4 out]
                n124 = Not(x=w410) -> (.not. x?=w409:bool)
                n125 = Greater?(x=w414, y=500) -> (0:w416:bool)
                n126 = Wait (ms)(milliseconds to wait=u32 1) -> ()  [unwired: 1 out]
                n127 = Or(x=w409, y=w416) -> (x .or. y?=w413:bool)
              }
              n128 = Index Array(array=w377, index #1=0 ("index"), index #2=1 ("index"), index #3=2 ("index")) -> (element #1=w376:T4, element #2=w375:T4, element #3=w374:T4)
              n129 = call "IMAQ Cast Image"("Image Type"=w399, "Image Dst"=w390, "Image Src"=w391) -> ("Image Dst Out"=w398:T4)  [unwired: 7 in, 1 out]
              n130 = call "4Pi Focus Lock - Norm FFT.vi"("FFT Image Dst"=w376, "Image In"=w398) -> ("FFT Image Out"=w387:T4)  [unwired: 8 in, 1 out]
              n131 = call "IMAQ ComplexConjugate"("Image Src"=w387) -> ("Image Dst Out"=w386:T4)  [unwired: 3 in, 1 out]
              n132 = for {
                tunnel: w372 -> [w408]
                tunnel: [w407] -> w397 mode=indexing
                tunnel: w386 -> [w406]
                tunnel: w389 -> [w405] mode=indexing
                tunnel: w374 -> [w404]
                tunnel: w375 -> [w403]
                n133 = call "4Pi Focus Lock - Get Cross Correlation.vi"("Ref FFT image"=w405, "Cur FFT Image"=w406, "FFT CC image"=w403, "iFFT image"=w404, "CC image"=w408) -> ("Max CC"=w407:sgl)  [unwired: 8 in, 2 out]
              }
              n134 = To Double Precision Float(number=w397) -> (double precision float=w388:dbl[])
              n135 = call "4Pi Focus Lock - Find Peak Position.vi"("Fit Size"=2, "y"=w388, "x"=w396) -> ("Coerced Peak Position"=w385:dbl)  [unwired: 6 in, 2 out]
              "Measured Z (µm)" <- w385
              n136 = Not A Number/Path/Refnum?(number/path/refnum=w385) -> (NaN/Path/Refnum?=w384:bool)
              n137 = Select(t=4Pi_Focus_Lock_-_Actions."Get Current Position", s=w384, f=4Pi_Focus_Lock_-_Actions."Check Drift" ("y")) -> (s? t:f=w381:T2)
            }
            frame "Get Current Position 1" {
              w435 = T5 2 items=["Grayscale (U8)", "Grayscale (I16)", "Grayscale (SGL)", "Complex (CSG)", "RGB (U32)", "HSL (U32)", "RGB (U64)", "Grayscale (U16)"] ("Image Type")
              n138 = Get Notifier Status(notifier=w436) -> (notifier out=w430:refnum<notifier>, current notification=w434:T3)  [unwired: 1 in, 3 out]
              n139 = Unbundle By Name(w434) -> ("Sample Z (µm)"=w433:dbl[])
              n140 = Unbundle By Name(w434) -> ("Ref Stack (SGL)"=w425:T4[])
              n141 = Unbundle By Name(w434) -> ("Cur Image (SGL)"=w426:T4, "CC Image (SGL)"=w421:T4)
              n142 = call "Camera Messenger.vi"("Notifier Name"=w437, "General Camera Actions"=Generic_Camera_Actions."Capture") -> ("Notifier Name Dup"=w428:string)  [unwired: 8 in, 5 out]
              n143 = while {
                tunnel: w428 -> [w458]
                tunnel: [w452] -> w427
                i -> [w454]
                stop <- w453 stop-if-true
                n144 = call "Camera Messenger.vi"("Notifier Name"=w458, "General Camera Actions"=Generic_Camera_Actions."Status") -> ("Running?"=w450:bool, "Image Ref"=w452:T4)  [unwired: 8 in, 4 out]
                n145 = Not(x=w450) -> (.not. x?=w449:bool)
                n146 = Greater?(x=w454, y=500) -> (0:w456:bool)
                n147 = Wait (ms)(milliseconds to wait=u32 1) -> ()  [unwired: 1 out]
                n148 = Or(x=w449, y=w456) -> (x .or. y?=w453:bool)
              }
              n149 = call "IMAQ Cast Image"("Image Type"=w435, "Image Dst"=w426, "Image Src"=w427) -> ("Image Dst Out"=w423:T4)  [unwired: 7 in, 1 out]
              n150 = call "4Pi Focus Lock - Img Norm.vi"("Image In"=w423) -> ("Image Dst Out"=w422:T4)  [unwired: 9 in, 1 out]
              n151 = for {
                tunnel: w425 -> [w448] mode=indexing
                tunnel: w422 -> [w446]
                tunnel: w421 -> [w445]
                tunnel: [w444] -> w420 mode=indexing
                n152 = call "4Pi Focus Lock - Img Norm.vi"("Image In"=w448) -> ("Image Dst Out"=w447:T4)  [unwired: 9 in, 1 out]
                n153 = call "IMAQ Multiply"("Image Src A"=w447, "Image Dst"=w445, "Image Src B"=w446) -> ("Image Dst Out"=w443:T4)  [unwired: 4 in, 1 out]
                n154 = call "IMAQ ImageToArray"("Image"=w443) -> ("Image Pixels (Float)"=w442:sgl[][])  [unwired: 3 in, 4 out]
                n155 = Add Array Elements(numeric array=w442) -> (sum=w440:sgl)
                n156 = Array Size(array=w442) -> (size(s)=w441:i32[])
                n157 = Multiply Array Elements(1:w441) -> (0:w439:i32)
                n158 = Divide(x=w440, y=w439) -> (x/y=w444:sgl)
              }
              n159 = To Double Precision Float(number=w420) -> (double precision float=w424:dbl[])
              n160 = call "4Pi Focus Lock - Find Peak Position.vi"("Fit Size"=2, "y"=w424, "x"=w433) -> ("Coerced Peak Position"=w419:dbl)  [unwired: 6 in, 2 out]
              n161 = local write "Measured Z (µm)"(w419) -> ()
            }
            frame "Check Drift" {
              n162 = Get Notifier Status(notifier=w470) -> (notifier out=w460:refnum<notifier>, current notification=w469:T3)  [unwired: 1 in, 3 out]
              n163 = local read "Measured Z (µm)"() -> (w471:dbl)
              n164 = Unbundle By Name(w469) -> ("Z Drift Threshold"=w463:dbl, "PID Values"=w468:dbl[])
              n165 = local read "Target Z (µm)"() -> (w472:dbl)
              n166 = Array To Cluster(array=w468) -> (cluster=w467:T12)
              n167 = call-poly <vilib>:"PID.vi"("PID gains"=w467, "process variable"=w471, "setpoint"=w472) -> ("dt out (s)"=→"dt (s)":dbl, "output"=w465:dbl)  [unwired: 7 in]
              "dz (µm)" <- w465
              n168 = Absolute Value(x=w465) -> (abs(x)=w464:dbl)
              n169 = Greater?(x=w464, y=w463) -> (0:→"Z Move":bool)
            }
            frame "Move Z" {
              n170 = Get Notifier Status(notifier=w488) -> (notifier out=w481:refnum<notifier>, current notification=w487:T3)  [unwired: 1 in, 3 out]
              n171 = Unbundle By Name(w487) -> ("Z Stage Move Limit (µm)"=w485:dbl)
              n172 = local read "dz (µm)"() -> (w486:dbl)
              n173 = Multiply(x=w486, y="Update Scale Factor") -> (x*y=w479:dbl)
              n174 = Absolute Value(x=w479) -> (abs(x)=w484:dbl)
              n175 = Greater?(x=w485, y=w484) -> (0:w475:bool)
              n176 = local read "Z Move"() -> (w477:bool)
              n177 = And(x=w475, y=w477) -> (x .and. y?=w478:bool)
              n178 = case shown="True" w478 {
                tunnel: w479 -> [_ w492]
                tunnel: w483 -> [_ w491]
                frame False {
                }
                frame True {
                  n179 = Build Array(w492) -> (w496:dbl[])
                  n180 = call "Stages Messenger.vi"("Stage Notifier Name"=w491, "Actions"=Stage_Actions."MVR", "Setpoint"=w496, "Axis"=bool[] [TRUE], "Exit While Busy?"=TRUE) -> ("Positions"=w494:dbl[])  [unwired: 7 in, 3 out]
                  n181 = Wait (ms)(milliseconds to wait=u32 50) -> ()  [unwired: 1 out]
                  n182 = Index Array(array=w494, index=0) -> ()  [unwired: 1 out]
                }
              }
              n183 = Select(t=4Pi_Focus_Lock_-_Actions."Update Plots" ("y"), s=w475, f=4Pi_Focus_Lock_-_Actions."Abort") -> (s? t:f=w473:T2)
            }
            frame "Update Plots" {
              n184 = Get Notifier Status(notifier=w512) -> (notifier out=w500:refnum<notifier>, current notification=w510:T3)  [unwired: 1 in, 3 out]
              n185 = Unbundle By Name(w510) -> ("Z Drift Threshold"=w511:dbl)
              n186 = Unbundle By Name(w510) -> ("Initial Z Position (µm)"=w509:dbl)
              n187 = call "Stages Messenger.vi"("Stage Notifier Name"=w502, "Actions"=Stage_Actions."Get Position", "Exit While Busy?"=TRUE) -> ("Positions"=w503:dbl[])  [unwired: 9 in, 3 out]
              n188 = local read "Measured Z (µm)"() -> (w513:dbl)
              n189 = local read "Target Z (µm)"() -> (w514:dbl)
              n190 = Index Array(array=w503, index=0) -> (element=w501:dbl)
              n191 = local write "Stage Position (µm)"(w501) -> ()
              n192 = Subtract(x=w501, y=w509) -> (x-y=w508:dbl)
              n193 = call "4Pi Focus Lock - Values Organize Plot Data.vi"("Target 01"=w514, "Value Limit"=w511, "Current 01"=w513, "Stage Position"=w508) -> ("output cluster"=→"Z Target and Fit Value (µm)":T1)  [unwired: 11 in]
            }
            frame "Abort" {
              n194 = Get Notifier Status(notifier=w520) -> (notifier out=w525:refnum<notifier>, current notification=w524:T3)  [unwired: 1 in, 3 out]
              n195 = call "Camera Messenger.vi"("Notifier Name"=w519, "General Camera Actions"=Generic_Camera_Actions."Abort") -> ()  [unwired: 8 in, 6 out]
              n196 = Bundle By Name(cluster=w524, "Running?"=FALSE, "Actions"=4Pi_Focus_Lock_-_Actions."Exit Loop") -> (w522:T3)
              n197 = Send Notification(notification=w522, notifier=w525) -> (notifier out=w516:refnum<notifier>)  [unwired: 1 in, 1 out]
            }
            frame "Exit Loop" {
            }
            frame "Quit" {
              n198 = Get Notifier Status(notifier=w530) -> (current notification=w536:T3)  [unwired: 1 in, 4 out]
              n199 = Unbundle By Name(w536) -> ("Ref Stack (SGL)"=w535:T4[], "Cur Image (SGL)"=w534:T4, "Tmp Image FFT (CSG)"=w533:T4[], "CC Image (SGL)"=w532:T4, "Ref FFT Stack (CSG)"=w529:T4[])
              n200 = Build Array (concatenate)(w535, w534, w533, w532, w529) -> (w531:T4[])
              n201 = for {
                tunnel: w531 -> [w539] mode=indexing
                n202 = call "IMAQ Dispose"("Image"=w539) -> ()  [unwired: 5 in, 1 out]
              }
            }
          }
          n203 = Get Notifier Status(notifier=w198) -> (current notification=w206:T3)  [unwired: 1 in, 4 out]
          n204 = Unbundle By Name(w206) -> ("Actions"=w205:T2)
          n205 = Equal?(x=w203, y=w205) -> (x = y?=w204:bool)
          n206 = Select(t=w203, s=w204, f=w202) -> (s? t:f=w201:T2)
        }
      }
      n207 = while {
        tunnel: w70 -> [w86]
        tunnel: w69 -> [w85]
        stop <- w84 stop-if-true
        n208 = event shown="[4] \"Start Lock\": Value Change" {
          selector: _ -> [_ _ _ _ _ _]
          dyn-events: _ -> [_ _ _ _ _ _]
          timeout: -1 -> [_ _ _ _ _ _]
          tunnel: w86 -> [_ w89 _ _ _ _]
          tunnel: w85 -> [_ _ w99 w136 w159 w163]
          tunnel: [w87 w88 w90 w132 w153 w161] -> w84
          tunnel: FALSE ("NewVal") -> [w87 w88 w90 w132 w153 _]
          event Timeout {
            n209 = event-data() -> ()  [unwired: 1 in, 3 out]
          }
          event "Set Camera ROI": Value Change {
            n210 = event-data() -> ()  [unwired: 1 in, 2 out]
            n211 = call "4Pi Focus Lock - Setup Camera.vi"("Camera Notifier Name"=w89) -> ()  [unwired: 14 in, 1 out]
          }
          event "P (Proportional)", "I (Integral)", "D (Derivative)", "Sample Z Step Size (µm)", "Z Move Limit (µm)", "Z Drift Threshold (µm)": Value Change {
            n212 = event-data() -> ("NewVal"=w94:dbl, "CtlRef"=w96:refnum<vi>)  [unwired: 1 in]
            n213 = Get Notifier Status(notifier=w99) -> (notifier out=w98:refnum<notifier>, current notification=w97:T3)  [unwired: 1 in, 3 out]
            n214 = property class="DigNum (strict)"(reference=w96) -> ("Label.Text"=w95:string)  [unwired: 1 in, 2 out]
            n215 = case shown="\"Z Drift Threshold (µm)\"" w95 {
              tunnel: w97 -> [w100 w103 w109 w115 w121 w124 w127]
              tunnel: w94 -> [_ w104 w110 w116 w120 w123 w126]
              tunnel: [w100 w101 w107 w113 w119 w122 w125] -> w93
              frame Default {
              }
              frame "P (Proportional)" {
                n216 = Unbundle By Name(w103) -> ("PID Values"=w105:dbl[])
                n217 = Replace Array Subset(array=w105, new element=w104, index=0) -> (w102:dbl[])
                n218 = Bundle By Name(cluster=w103, "PID Values"=w102) -> (w101:T3)
              }
              frame "I (Integral)" {
                n219 = Unbundle By Name(w109) -> ("PID Values"=w111:dbl[])
                n220 = Replace Array Subset(array=w111, new element=w110, index=1) -> (w108:dbl[])
                n221 = Bundle By Name(cluster=w109, "PID Values"=w108) -> (w107:T3)
              }
              frame "D (Derivative)" {
                n222 = Unbundle By Name(w115) -> ("PID Values"=w117:dbl[])
                n223 = Replace Array Subset(array=w117, new element=w116, index=2) -> (w114:dbl[])
                n224 = Bundle By Name(cluster=w115, "PID Values"=w114) -> (w113:T3)
              }
              frame "Sample Z Step Size (µm)" {
                n225 = Bundle By Name(cluster=w121, "Z Step Size (µm)"=w120) -> (w119:T3)
              }
              frame "Z Move Limit (µm)" {
                n226 = Bundle By Name(cluster=w124, "Z Stage Move Limit (µm)"=w123) -> (w122:T3)
              }
              frame "Z Drift Threshold (µm)" {
                n227 = Bundle By Name(cluster=w127, "Z Drift Threshold"=w126) -> (w125:T3)
              }
            }
            n228 = Bundle By Name(cluster=w93, "Actions"=4Pi_Focus_Lock_-_Actions."Idle") -> (w91:T3)
            n229 = Send Notification(notification=w91, notifier=w98) -> ()  [unwired: 1 in, 2 out]
          }
          event "Sample Z Step No.": Value Change {
            n230 = event-data() -> ("NewVal"=w130:u32)  [unwired: 1 in]
            n231 = Get Notifier Status(notifier=w136) -> (notifier out=w134:refnum<notifier>, current notification=w135:T3)  [unwired: 1 in, 3 out]
            n232 = for {
              N: w130 -> [_]
              tunnel: [w148] -> w129 mode=indexing
              tunnel: [w137] -> w128 mode=indexing
              i -> [w147]
              w138 = T5 3 items=["Grayscale (U8)", "Grayscale (I16)", "Grayscale (SGL)", "Complex (CSG)", "RGB (U32)", "HSL (U32)", "RGB (U64)", "Grayscale (U16)"] ("Image Type")
              w143 = T5 2 items=["Grayscale (U8)", "Grayscale (I16)", "Grayscale (SGL)", "Complex (CSG)", "RGB (U32)", "HSL (U32)", "RGB (U64)", "Grayscale (U16)"] ("Image Type")
              w139 = 10 ("Border Size")
              n233 = Number To Decimal String(number=w147, width (-)=i16 1) -> (decimal integer string=w145:string)
              n234 = Concatenate Strings("Ref Stack " ("string"), w145) -> (w141:string)
              n235 = call "IMAQ Create"("Border Size"=w139, "Image Name"=w141, "Image Type"=w143) -> ("New Image"=w148:T4)  [unwired: 2 in, 1 out]
              n236 = Concatenate Strings("FFT" ("string"), w141) -> (w140:string)
              n237 = call "IMAQ Create"("Border Size"=w139, "Image Name"=w140, "Image Type"=w138) -> ("New Image"=w137:T4)  [unwired: 2 in, 1 out]
            }
            n238 = Bundle By Name(cluster=w135, "Actions"=4Pi_Focus_Lock_-_Actions."Idle", "Z Step No."=w130, "Ref Stack (SGL)"=w129, "Ref FFT Stack (CSG)"=w128) -> (w133:T3)
            n239 = Send Notification(notification=w133, notifier=w134) -> ()  [unwired: 1 in, 2 out]
          }
          event "Start Lock": Value Change {
            n240 = event-data() -> ("NewVal"=w151:bool)  [unwired: 1 in]
            n241 = Select(t=4Pi_Focus_Lock_-_Actions."Start Lock", s=w151, f=4Pi_Focus_Lock_-_Actions."Abort" ("t")) -> (s? t:f=w156:T2)
            n242 = Select(t=TRUE ("Running?"), s=w151, f=FALSE) -> (s? t:f=w149:bool)
            n243 = Get Notifier Status(notifier=w159) -> (notifier out=w160:refnum<notifier>, current notification=w158:T3)  [unwired: 1 in, 3 out]
            n244 = Bundle By Name(cluster=w158, "Actions"=w156, "Running?"=w149) -> (w157:T3)
            n245 = Send Notification(notification=w157, notifier=w160) -> ()  [unwired: 1 in, 2 out]
          }
          event "Quit": Value Change {
            # "Turn off the Focus lock before quiting."
            n246 = event-data() -> ("NewVal"=w161:bool)  [unwired: 1 in]
            n247 = Get Notifier Status(notifier=w163) -> (notifier out=w166:refnum<notifier>, current notification=w164:T3)  [unwired: 1 in, 3 out]
            n248 = Unbundle By Name(w164) -> ("Running?"=w167:bool)
            n249 = case shown="False" w167 {
              tunnel: w166 -> [w171 w176]
              tunnel: [w171 w173] -> w165
              tunnel: w164 -> [_ w177]
              frame False {
              }
              frame True {
                n250 = Bundle By Name(cluster=w177, "Actions"=4Pi_Focus_Lock_-_Actions."Abort") -> (w175:T3)
                n251 = Send Notification(notification=w175, notifier=w176) -> (notifier out=w174:refnum<notifier>)  [unwired: 1 in, 1 out]
                n252 = while {
                  tunnel: w174 -> [w187]
                  tunnel: [w182] -> w173
                  i -> [w181]
                  stop <- w183 stop-if-true
                  n253 = Get Notifier Status(notifier=w187) -> (notifier out=w182:refnum<notifier>, # waiting=w186:i32)  [unwired: 1 in, 3 out]
                  n254 = Greater?(x=w181, y=1500) -> (0:w179:bool)
                  n255 = Less?(x=w186, y=1) -> (x < y?=w184:bool)
                  n256 = Or(x=w184, y=w179) -> (x .or. y?=w183:bool)
                  n257 = Wait (ms)(milliseconds to wait=u32 1) -> ()  [unwired: 1 out]
                }
              }
            }
            n258 = Get Notifier Status(notifier=w165) -> (notifier out=w169:refnum<notifier>, current notification=w170:T3)  [unwired: 1 in, 3 out]
            n259 = Bundle By Name(cluster=w170, "Actions"=4Pi_Focus_Lock_-_Actions."Quit") -> (w168:T3)
            n260 = Send Notification(notification=w168, notifier=w169) -> ()  [unwired: 1 in, 2 out]
          }
        }
      }
      n261 = Release Notifier(notifier=w67, force destroy? (F)=TRUE) -> ()  [unwired: 1 in, 3 out]
    }
    frame Error {
    }
  }
